vi "configuration UI.vi"() -> ()   [LabVIEW 2013, in "OPC UA Client editor node.lvclass"]
uses:
  OPC UA Client editor node.lvclass
  <vilib>/NI/Configuration Framework/Node/NodeRef.ctl
  <vilib>/NI/Configuration Framework/Node/NISE_CEF_Node.lvclass
  <vilib>/NI/AMC/Message Queue.ctl
  <vilib>/NI/AMC/Message.ctl
  <vilib>/NI/Tools/Keyed Array/KeyedArray.ctl
  <vilib>/NI/Configuration Framework/Node/UserEventRef.ctl
  <vilib>/NI/Configuration Framework/Controls/EventCluster.ctl
  <vilib>/NI/DCAF UI Toolkit/Controls/Configure.ctl
  <vilib>/NI/DCAF UI Toolkit/Controls/Add.ctl
  <vilib>/NI/DCAF UI Toolkit/Controls/Remove.ctl
  <vilib>/NI/Configuration Framework/Node/StopEvent.ctl
  <vilib>/NI/Configuration Framework/Node/RefreshUIEvent.ctl
  <vilib>/NI/Configuration Framework/Node/CacheState.ctl
  <vilib>/NI/Configuration Framework/Node/NodeChangeEvent.ctl
  <vilib>/NI/Tag Bus/tag/Data Type.ctl
  Permissions Enum.ctl
  <vilib>/NI/DCAF/Tag Editor Core/Table API/Available Tag Menu/channel action event.ctl
  <vilib>/NI/DCAF/Tag Editor Core/Table API/Available Tag Menu/dialog output action.ctl
  <vilib>/NI/Tag Bus Module Framework/channel/TBM channel.lvclass
  <vilib>/NI/Tag Bus/tag/tag descriptor.lvclass
  <vilib>/NI/DCAF/Tag Editor Core/Table API/Table Manager/Call Back Ref Type Def.ctl
  <vilib>/NI/DCAF/Tag Editor Core/Configuration Editor/Classes/Engine Parent/Engine Parent Editor Node.lvclass
  OPC UA DataType Enum.ctl
  <vilib>/NI/DCAF/Tag Editor Core/Table API/Table Manager/references.ctl
  module/configuration/OPC UA Client configuration.lvclass
  module/configuration/OPC UA Client configuration.lvclass/OPC UA Client configuration.ctl
  <vilib>/NI/DCAF/Tag Editor Core/Table API/Listbox/Multi Column Listbox.lvclass
  OPC UA Client editor node.lvclass/OPC UA Client editor node.ctl
  module/configuration/Read Connection Configuration.vi
  module/configuration/Write Connection Configuration.vi
  <vilib>/NI/DCAF/Tag Editor Core/Configuration Editor/Classes/Module editor node/module editor node.lvclass
  <vilib>/NI/Configuration Framework/serializable configuration/NISE_CEF_serializable configuration.lvclass
  <vilib>/NI/Configuration Framework/NISE_CEF_TreeControl.lvlib
  <vilib>/NI/Tools/Keyed Array/Tools_KeyedArray.lvlib
  <vilib>/NI/AMC/AMC.lvlib
  <vilib>/NI/DCAF/Tag Editor Core/Table API/Table Manager.lvlib
  <vilib>/NI/DCAF/Tag Editor Core/Table API/Table Manager/Table Manager.lvclass
  <vilib>/NI/DCAF UI Toolkit/Controls/DCAF UI Elements.lvlib
panel:
  in  "OPC Data Type":T1
  in  "user event out":refnum<user-event>
  in  "Permissions":T2
  in  "data type":T3
  in  "node change":T4
  in  "cache state":T5
  in  "refresh UI":T6
  in  "stop event":T7
  in  "Tab Control":enum32{"Nodes", "Client Configuration"}(tab)
  in  "Remove Button":T8
  in  "Add Button":T9
  in  "Table":i32(listbox)
  in  "settings":T10
  in  "Server Certificates":path[](array[path])
  in  "Client Certificate":path
  in  "Server Endpoint URL":string
  in  "Username/Password":cluster{"Username":string, "Password":string}
  in  "Security Policy":T11
  in  "user event":T12
  in  "main queue":T13
  in  "node ref":T14
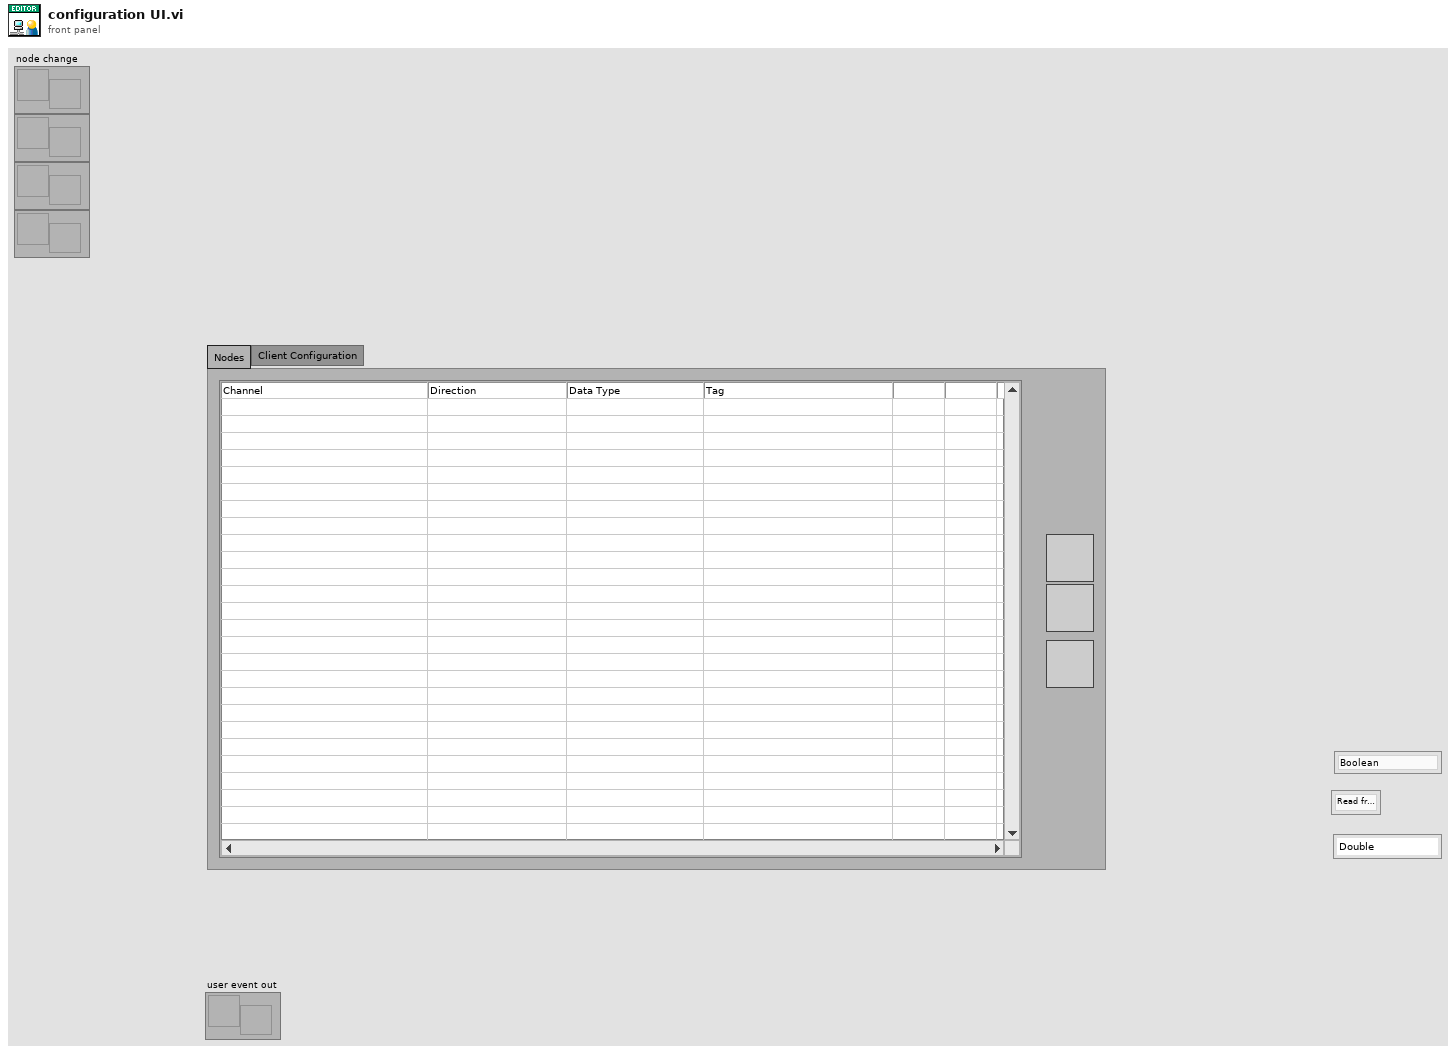
[diagram p1: front panel]
types:
  T1 = typedef "OPC UA Client editor node.lvclass/OPC UA DataType Enum.ctl" = enum16{"Boolean", "SByte", "Byte", "Int16", "UInt16", "Int32", "UInt32", "Int64", "UInt64", "Float", "Double", "String", "DateTime", "ByteString", "Array of Boolean", "Array of SByte", "Array of Byte", "Array of Int16", "Array of UInt16", "Array of Int32", "Array of UInt32", "Array of Int64", "Array of UInt64", "Array of Float", "Array of Double", "Array of String", "Array of DateTime"}
  T2 = typedef "OPC UA Client editor node.lvclass/Permissions Enum.ctl" = enum16{"Read from HW", "Write to HW"}
  T3 = typedef "tag bus.lvlib/tag descriptor.lvclass/Data Type.ctl" = enum16{"Double", "Single", "I64", "I32", "I16", "I8", "U64", "U32", "U16", "U8", "Boolean", "String", "Array of Double", "Array of Single", "Array of I64", "Array of I32", "Array of I16", "Array of I8", "Array of U64", "Array of U32", "Array of U16", "Array of U8", "Array of Boolean", "Array of String"}
  T4 = typedef "NISE_CEF_Node.lvclass/NodeChangeEvent.ctl" = refnum<user-event>
  T5 = typedef "NISE_CEF_Node.lvclass/CacheState.ctl" = refnum<user-event>
  T6 = typedef "NISE_CEF_Node.lvclass/RefreshUIEvent.ctl" = refnum<user-event>
  T7 = typedef "NISE_CEF_Node.lvclass/StopEvent.ctl" = refnum<user-event>
  T8 = typedef "DCAF UI Elements.lvlib/Remove.ctl" = bool
  T9 = typedef "DCAF UI Elements.lvlib/Add.ctl" = bool
  T10 = typedef "DCAF UI Elements.lvlib/Configure.ctl" = bool
  T11 = cluster{"Message Mode":enum16{"None", "Sign", "Sign and Encrypt"}, "Security":enum16{"Basic256", "Basic128Rsa15"}}
  T12 = typedef "NISE_CEF_Node.lvclass/UserEventRef.ctl" = refnum<user-event>
  T13 = typedef "AMC.lvlib/Message Queue.ctl" = refnum<queue>
  T14 = typedef "NISE_CEF_Node.lvclass/NodeRef.ctl" = refnum<data-value>
  T15 = typedef "Table Manager.lvlib/Table Manager.lvclass/references.ctl" = cluster{"stop event":T7, "refresh UI":T6, "cache state":T5, "node change":T4, "user event out":refnum<user-event>, "main queue":T13, "user event":T12}
  T16 = typedef "Table Manager.lvlib/Table Manager.lvclass/object ref.ctl" = cluster{"engine":refnum<data-value>, "Node Ref":refnum<data-value>}
  T17 = cluster{"Server Certificates":cluster{"Relative Path?":bool, "Certificate Paths":path[], "Certificate Names":string[]}, "Client Certificates":cluster{"Relative Path?":bool, "Certificate Paths":path[], "Certificate Names":string[]}, "Client Configuration":cluster{"Server Endpoint URL":string, "Security Policy":cluster{"Message Mode":enum16{"None", "Sign", "Sign and Encrypt"}, "Security":enum16{"Basic256", "Basic128Rsa15"}}, "Username/Password":cluster{"Username":string, "Password":string}}}
  T18 = typedef "Table Manager.lvlib/Column.lvclass/Column Descriptor.ctl" = cluster{"name":string, "caption":string, "Column Type":T19, "Params":string, "AutoSizeMode":i32, "FillWeight":sgl, "MinWidth":u32, "tooltip":string, "Enum Reference":refnum<vi>, "Channel suffix":string, "Read Only":bool, "Call Back VI":T20, "DT Dependency":i32, "name dependency":i32, "data type":T3, "Custom Column":refnum<class "Column.lvclass">}
  T19 = typedef "Table Manager.lvlib/Column.lvclass/Column Type.ctl" = enum16{"String", "Mapping", "Enum", "Custom"}
  T20 = typedef "Table Manager.lvlib/Table Manager.lvclass/Call Back Ref Type Def.ctl" = refnum<vi>
  T21 = typedef "Table Manager.lvlib/Table Manager.lvclass/Table Events.ctl" = cluster{"Menu Selection":refnum<user-event>}
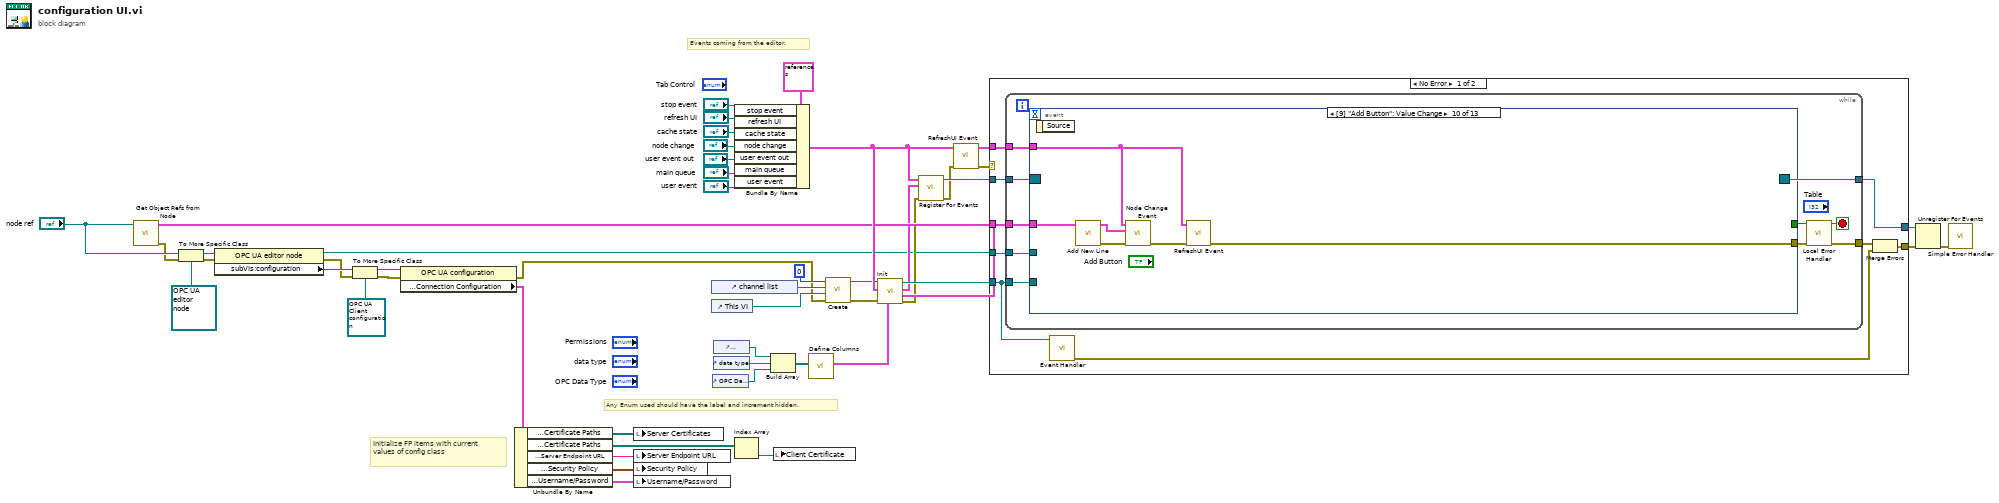
[diagram p0: block diagram]
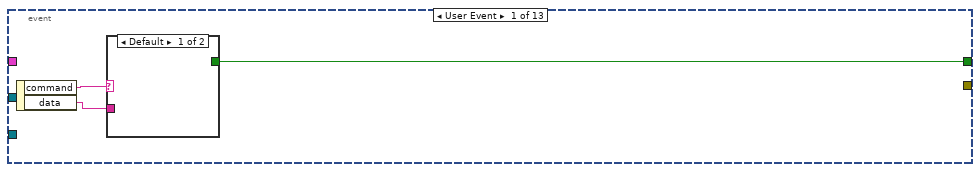
[diagram p2: hidden frame]
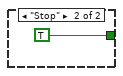
[diagram p3: hidden frame]
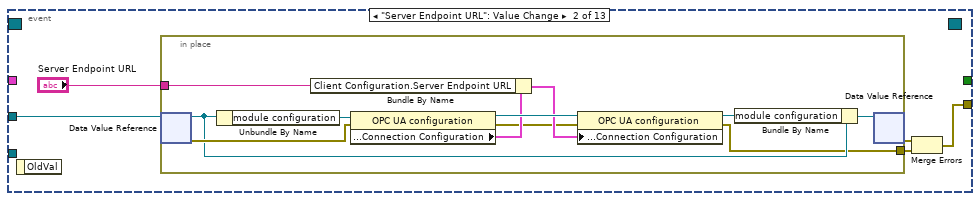
[diagram p4: hidden frame]
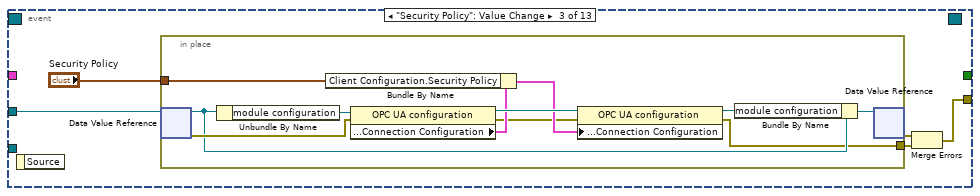
[diagram p5: hidden frame]
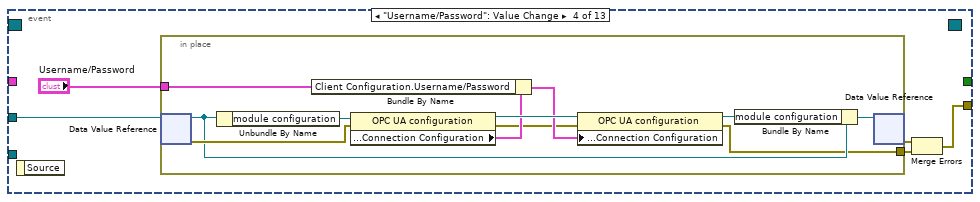
[diagram p6: hidden frame]
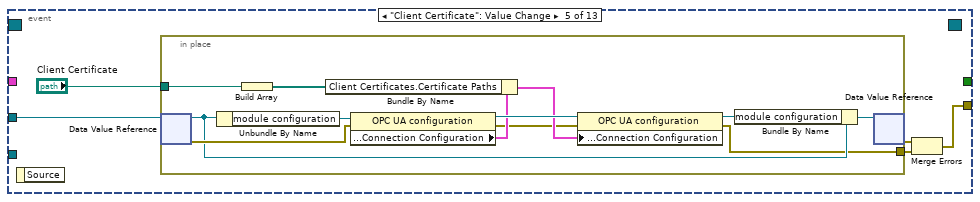
[diagram p7: hidden frame]
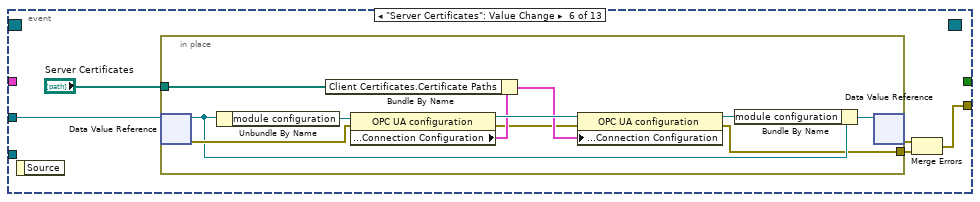
[diagram p8: hidden frame]
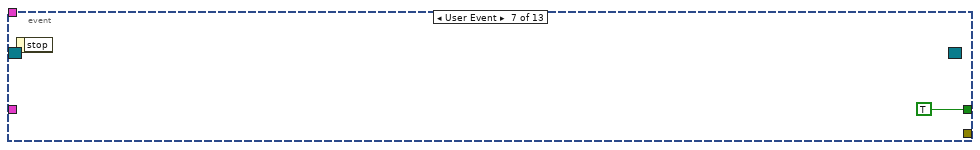
[diagram p9: hidden frame]
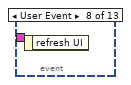
[diagram p10: hidden frame]
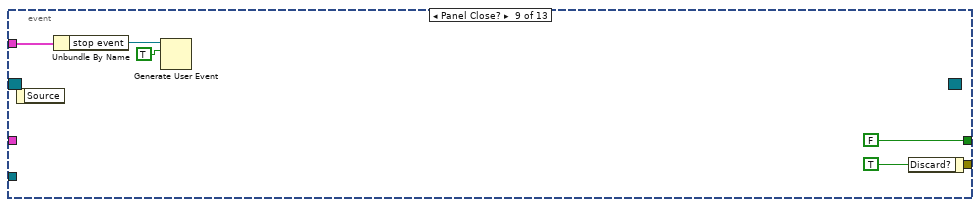
[diagram p11: hidden frame]
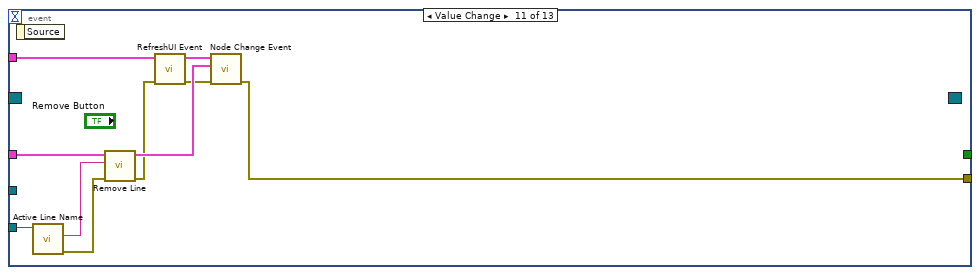
[diagram p12: hidden frame]
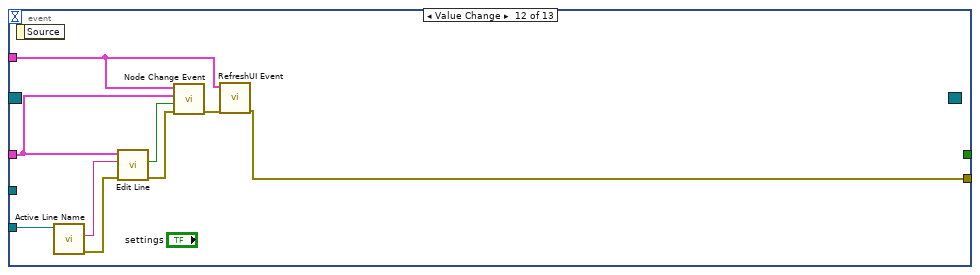
[diagram p13: hidden frame]
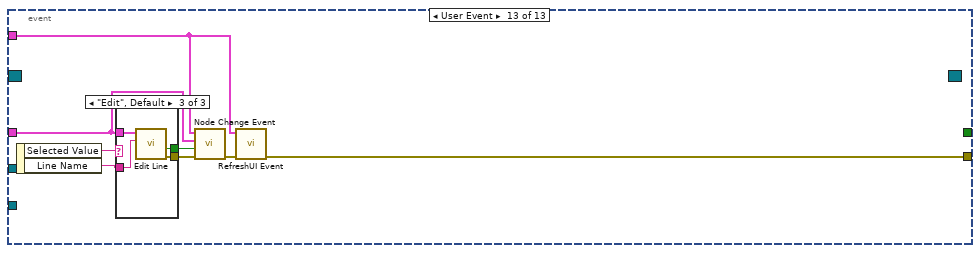
[diagram p14: hidden frame]
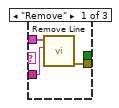
[diagram p15: hidden frame]
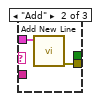
[diagram p16: hidden frame]
diagram:
  # "Initialize FP items with current values of config class"
  # "Any Enum used should have the label and increment hidden."
  # "Events coming from the editor."
  n1 = call "Get Object Refs from Node.vi"("Data Value Reference in"="node ref") -> ("error out"=w18:errorcluster, "references"=w32:T16)  [unwired: 9 in]
  n2 = To More Specific Class(target class=refnum<data-value> refnum ("data value reference"), reference="node ref", error in=w18) -> (specific class reference=w16:refnum<data-value>, error out=w17:errorcluster)
  n3 = property class="OPC UA editor node"(reference=w16, error in=w17) -> (reference out=w15:refnum<data-value>, error out=w9:errorcluster, "subVIs:configuration"=w14:refnum<class "NISE_CEF_serializable configuration.lvclass">)
  n4 = To More Specific Class(target class=refnum<class "OPC UA Client configuration.lvclass"> refnum ("OPC UA configuration"), reference=w14, error in=w9) -> (specific class reference=w13:refnum<class "OPC UA Client configuration.lvclass">, error out=w12:errorcluster)
  n5 = property class="OPC UA configuration"(reference=w13, error in=w12) -> (error out=w8:errorcluster, "Customize:Properties:Connection Configuration"=w10:T17)  [unwired: 1 out]
  n6 = Unbundle By Name(w10) -> ("Server Certificates.Certificate Paths"=w6:path[], "Client Certificates.Certificate Paths"=w5:path[], "Client Configuration.Server Endpoint URL"=w1:string, "Client Configuration.Security Policy"=w2:T11, "Client Configuration.Username/Password"=w3:cluster{"Username":string, "Password":string})
  n7 = local write "Server Certificates"(w6) -> ()
  n8 = local write "Server Endpoint URL"(w1) -> ()
  n9 = local write "Security Policy"(w2) -> ()
  n10 = local write "Username/Password"(w3) -> ()
  n11 = control-ref of="channel list"() -> (w25:refnum<vi>)
  n12 = control-ref of="This VI"() -> (w23:refnum<vi>)
  n13 = control-ref of="OPC Data Type"() -> (w21:refnum<vi>)
  n14 = control-ref of="Permissions"() -> (w35:refnum<vi>)
  n15 = control-ref of="data type"() -> (w34:refnum<vi>)
  n16 = Bundle By Name(cluster=T15 {"stop event"=refnum, "refresh UI"=refnum, "cache state"=refnum, "node change"=refnum, "user event out"=refnum, "main queue"=refnum, "user event"=refnum} ("References"), "stop event"="stop event", "refresh UI"="refresh UI", "cache state"="cache state", "node change"="node change", "user event out"="user event out", "main queue"="main queue", "user event"="user event") -> (w36:T15)
  n17 = Index Array(array=w5) -> (element=w4:path)  [unwired: 1 in]
  n18 = Build Array(w35, w34, w21) -> (w33:refnum<vi>[])
  n19 = local write "Client Certificate"(w4) -> ()
  n20 = call "Define Columns.vi"("Enum Array"=w33) -> ("Column Definition"=w38:T18[])  [unwired: 10 in]
  n21 = call <vilib>:"Create.vi"("error in (no error)"=w8, "Top VI"=w23, "Listbox"=w25, "Index"=0) -> ("error out"=w7:errorcluster, "reference out"=w22:refnum<class "Multi Column Listbox.lvclass">)  [unwired: 6 in]
  n22 = call-dynamic "Init.vi"("Column Descriptors"=w38, "error in (no error)"=w7, "Node object refs"=w32, "Event References"=w36, "Multi Column Listbox in"=w22) -> ("error out"=w27:errorcluster, "Table Events"=w26:T21, "Multi Column Listbox out"=w31:refnum<class "Multi Column Listbox.lvclass">)  [unwired: 4 in]
  n23 = call "Register For Events.vi"("error in"=w27, "Table Events"=w26, "References"=w36) -> ("error out"=w29:errorcluster, "Event Registration Refnum"=w39:refnum<event-registration>)  [unwired: 7 in]
  n24 = call "RefreshUI Event.vi"("error in (no error)"=w29, "References in"=w36) -> ("error out"=w28:errorcluster, "References out"=w37:T15)  [unwired: 8 in]
  n25 = case shown="No Error" w28 {
    selector: w28 -> [_ w201]
    tunnel: w39 -> [w58 w200]
    tunnel: [w57 w200] -> w49
    tunnel: [w51 w201] -> w48
    tunnel: w37 -> [w56 _]
    tunnel: w32 -> [w55 _]
    tunnel: w31 -> [w54 _]
    tunnel: w15 -> [w50 _]
    frame No Error {
      n26 = while {
        tunnel: w58 -> [w68]
        tunnel: [w67] -> w57
        tunnel: [w64] -> w52
        tunnel: w56 -> [w62]
        tunnel: w55 -> [w61]
        tunnel: w54 -> [w60]
        tunnel: w50 -> [w59]
        stop <- w66 stop-if-true
        n27 = event shown="[9] \"Add Button\": Value Change" {
          selector: w68 -> [_ _ _ _ _ _ _ _ _ _ _ _ _]
          dyn-events: [_ _ _ _ _ _ _ _ _ _ _ _ _] -> w67
          timeout: _ -> [_ _ _ _ _ _ _ _ _ _ _ _ _]
          tunnel: [w71 _ _ _ _ _ TRUE _ FALSE _ _ _ _] -> w65
          tunnel: [_ w73 w90 w106 w122 w139 _ _ _ w160 w168 w175 w188] -> w63
          tunnel: w62 -> [_ _ _ _ _ _ _ _ w156 w163 w173 w174 w184]
          tunnel: w61 -> [_ _ _ _ _ _ _ _ _ w164 w172 w180 w185]
          tunnel: w60 -> [_ _ _ _ _ _ _ _ _ _ w167 w181 _]
          tunnel: w59 -> [_ w77 w93 w109 w125 w142 _ _ _ _ _ _ _]
          event User Event {
            n28 = event-data() -> ("command"=w70:string, "data"=w69:string)  [unwired: 1 in]
            n29 = case shown="Default" w70 {
              tunnel: [_ TRUE] -> w71
              tunnel: w69 -> [_ _]
              frame Default {
              }
              frame "Stop" {
              }
            }
          }
          event "Server Endpoint URL": Value Change {
            n30 = event-data() -> ()  [unwired: 1 in, 1 out]
            n31 = in-place {
              in-place-border: "Server Endpoint URL" -> [w84]
              in-place-border: [w78] -> w74
              n32 = in-place-dvr #1(w77) -> (w80:refnum<class "OPC UA Client editor node.lvclass">, w83:errorcluster)
              n33 = Unbundle By Name(w80) -> ("module configuration"=w88:refnum<class "OPC UA Client configuration.lvclass">)
              n34 = property class="OPC UA configuration"(reference=w88, error in=w83) -> (reference out=w87:refnum<class "OPC UA Client configuration.lvclass">, error out=w82:errorcluster, "Customize:Properties:Connection Configuration"=w86:T17)
              n35 = Bundle By Name(cluster=w86, "Client Configuration.Server Endpoint URL"=w84) -> (w85:T17)
              n36 = property class="OPC UA configuration"(reference=w87, error in=w82, "Customize:Properties:Connection Configuration"=w85) -> (reference out=w81:refnum<class "OPC UA Client configuration.lvclass">, error out=w78:errorcluster)
              n37 = Bundle By Name(cluster=w80, "module configuration"=w81) -> (w79:refnum<class "OPC UA Client editor node.lvclass">)
              n38 = in-place-dvr #1(w79) -> (w75:errorcluster)  [unwired: 1 out]
            }
            n39 = Merge Errors(w75, w74) -> (w73:errorcluster)
          }
          event "Security Policy": Value Change {
            n40 = event-data() -> ()  [unwired: 1 in, 1 out]
            n41 = in-place {
              in-place-border: "Security Policy" -> [w100]
              in-place-border: [w94] -> w91
              n42 = in-place-dvr #2(w93) -> (w96:refnum<class "OPC UA Client editor node.lvclass">, w99:errorcluster)
              n43 = Unbundle By Name(w96) -> ("module configuration"=w104:refnum<class "OPC UA Client configuration.lvclass">)
              n44 = property class="OPC UA configuration"(reference=w104, error in=w99) -> (reference out=w103:refnum<class "OPC UA Client configuration.lvclass">, error out=w98:errorcluster, "Customize:Properties:Connection Configuration"=w102:T17)
              n45 = Bundle By Name(cluster=w102, "Client Configuration.Security Policy"=w100) -> (w101:T17)
              n46 = property class="OPC UA configuration"(reference=w103, error in=w98, "Customize:Properties:Connection Configuration"=w101) -> (reference out=w97:refnum<class "OPC UA Client configuration.lvclass">, error out=w94:errorcluster)
              n47 = Bundle By Name(cluster=w96, "module configuration"=w97) -> (w95:refnum<class "OPC UA Client editor node.lvclass">)
              n48 = in-place-dvr #2(w95) -> (w92:errorcluster)  [unwired: 1 out]
            }
            n49 = Merge Errors(w92, w91) -> (w90:errorcluster)
          }
          event "Username/Password": Value Change {
            n50 = event-data() -> ()  [unwired: 1 in, 1 out]
            n51 = in-place {
              in-place-border: "Username/Password" -> [w116]
              in-place-border: [w110] -> w107
              n52 = in-place-dvr #3(w109) -> (w112:refnum<class "OPC UA Client editor node.lvclass">, w115:errorcluster)
              n53 = Unbundle By Name(w112) -> ("module configuration"=w120:refnum<class "OPC UA Client configuration.lvclass">)
              n54 = property class="OPC UA configuration"(reference=w120, error in=w115) -> (reference out=w119:refnum<class "OPC UA Client configuration.lvclass">, error out=w114:errorcluster, "Customize:Properties:Connection Configuration"=w118:T17)
              n55 = Bundle By Name(cluster=w118, "Client Configuration.Username/Password"=w116) -> (w117:T17)
              n56 = property class="OPC UA configuration"(reference=w119, error in=w114, "Customize:Properties:Connection Configuration"=w117) -> (reference out=w113:refnum<class "OPC UA Client configuration.lvclass">, error out=w110:errorcluster)
              n57 = Bundle By Name(cluster=w112, "module configuration"=w113) -> (w111:refnum<class "OPC UA Client editor node.lvclass">)
              n58 = in-place-dvr #3(w111) -> (w108:errorcluster)  [unwired: 1 out]
            }
            n59 = Merge Errors(w108, w107) -> (w106:errorcluster)
          }
          event "Client Certificate": Value Change {
            n60 = event-data() -> ()  [unwired: 1 in, 1 out]
            n61 = in-place {
              in-place-border: "Client Certificate" -> [w133]
              in-place-border: [w127] -> w123
              n62 = in-place-dvr #4(w125) -> (w129:refnum<class "OPC UA Client editor node.lvclass">, w132:errorcluster)
              n63 = Unbundle By Name(w129) -> ("module configuration"=w137:refnum<class "OPC UA Client configuration.lvclass">)
              n64 = Build Array(w133) -> (w126:path[])
              n65 = property class="OPC UA configuration"(reference=w137, error in=w132) -> (reference out=w136:refnum<class "OPC UA Client configuration.lvclass">, error out=w131:errorcluster, "Customize:Properties:Connection Configuration"=w135:T17)
              n66 = Bundle By Name(cluster=w135, "Client Certificates.Certificate Paths"=w126) -> (w134:T17)
              n67 = property class="OPC UA configuration"(reference=w136, error in=w131, "Customize:Properties:Connection Configuration"=w134) -> (reference out=w130:refnum<class "OPC UA Client configuration.lvclass">, error out=w127:errorcluster)
              n68 = Bundle By Name(cluster=w129, "module configuration"=w130) -> (w128:refnum<class "OPC UA Client editor node.lvclass">)
              n69 = in-place-dvr #4(w128) -> (w124:errorcluster)  [unwired: 1 out]
            }
            n70 = Merge Errors(w124, w123) -> (w122:errorcluster)
          }
          event "Server Certificates": Value Change {
            n71 = event-data() -> ()  [unwired: 1 in, 1 out]
            n72 = in-place {
              in-place-border: "Server Certificates" -> [w149]
              in-place-border: [w143] -> w140
              n73 = in-place-dvr #5(w142) -> (w145:refnum<class "OPC UA Client editor node.lvclass">, w148:errorcluster)
              n74 = Unbundle By Name(w145) -> ("module configuration"=w153:refnum<class "OPC UA Client configuration.lvclass">)
              n75 = property class="OPC UA configuration"(reference=w153, error in=w148) -> (reference out=w152:refnum<class "OPC UA Client configuration.lvclass">, error out=w147:errorcluster, "Customize:Properties:Connection Configuration"=w151:T17)
              n76 = Bundle By Name(cluster=w151, "Client Certificates.Certificate Paths"=w149) -> (w150:T17)
              n77 = property class="OPC UA configuration"(reference=w152, error in=w147, "Customize:Properties:Connection Configuration"=w150) -> (reference out=w146:refnum<class "OPC UA Client configuration.lvclass">, error out=w143:errorcluster)
              n78 = Bundle By Name(cluster=w145, "module configuration"=w146) -> (w144:refnum<class "OPC UA Client editor node.lvclass">)
              n79 = in-place-dvr #5(w144) -> (w141:errorcluster)  [unwired: 1 out]
            }
            n80 = Merge Errors(w141, w140) -> (w139:errorcluster)
          }
          event User Event {
            n81 = event-data() -> ()  [unwired: 1 in, 1 out]
          }
          event User Event {
            n82 = event-data() -> ()  [unwired: 1 in, 1 out]
          }
          event Panel Close? {
            n83 = event-data() -> ()  [unwired: 1 in, 1 out]
            n84 = Unbundle By Name(w156) -> ("stop event"=w155:T7)
            n85 = Generate User Event(user event=w155, event data cluster=TRUE ("event data")) -> ()  [unwired: 2 in, 2 out]
            n86 = event-data("Discard?"=TRUE) -> ()  [unwired: 1 in, 1 out]
          }
          event Value Change {
            n87 = event-data() -> ()  [unwired: 1 in, 1 out]
            n88 = call "Add New Line.vi"("objects"=w164) -> ("error out"=w162:errorcluster)  [unwired: 9 in, 1 out]
            n89 = call "Node Change Event.vi"("error in (no error)"=w162, "objects"=w164, "References in"=w163) -> ("error out"=w161:errorcluster)  [unwired: 8 in]
            n90 = call "RefreshUI Event.vi"("error in (no error)"=w161, "References in"=w163) -> ("error out"=w160:errorcluster)  [unwired: 8 in, 1 out]
          }
          event Value Change {
            n91 = event-data() -> ()  [unwired: 1 in, 1 out]
            n92 = call-dynamic "Active Line Name.vi"("Multi Column Listbox in"=w167) -> ("error out"=w165:errorcluster, "Active Line Name"=w166:string)  [unwired: 8 in, 1 out]
            n93 = call "Remove Line.vi"("error in"=w165, "Active Line Name"=w166, "Objects"=w172) -> ("error out"=w169:errorcluster)  [unwired: 8 in]
            n94 = call "RefreshUI Event.vi"("error in (no error)"=w169, "References in"=w173) -> ("error out"=w171:errorcluster, "References out"=w170:T15)  [unwired: 8 in]
            n95 = call "Node Change Event.vi"("error in (no error)"=w171, "objects"=w172, "References in"=w170) -> ("error out"=w168:errorcluster)  [unwired: 8 in]
          }
          event Value Change {
            n96 = event-data() -> ()  [unwired: 1 in, 1 out]
            n97 = call-dynamic "Active Line Name.vi"("Multi Column Listbox in"=w181) -> ("error out"=w178:errorcluster, "Active Line Name"=w179:string)  [unwired: 8 in, 1 out]
            n98 = call "Edit Line.vi"("error in"=w178, "Line Name"=w179, "References"=w180) -> ("error out"=w182:errorcluster, "change?"=w177:bool)  [unwired: 7 in]
            n99 = call "Node Change Event.vi"("error in (no error)"=w182, "Send"=w177, "objects"=w180, "References in"=w174) -> ("error out"=w176:errorcluster)  [unwired: 7 in]
            n100 = call "RefreshUI Event.vi"("error in (no error)"=w176, "References in"=w174) -> ("error out"=w175:errorcluster)  [unwired: 8 in, 1 out]
          }
          event User Event {
            n101 = event-data() -> ("Selected Value"=w190:string, "Line Name"=w187:string)  [unwired: 1 in]
            n102 = case shown="\"Edit\", Default" w190 {
              tunnel: w187 -> [w193 _ w199]
              tunnel: w185 -> [w192 w195 w198]
              tunnel: [w191 w194 w197] -> w186
              tunnel: [_ _ w196] -> w183
              frame "Remove" {
                n103 = call "Remove Line.vi"("Active Line Name"=w193, "Objects"=w192) -> ("error out"=w191:errorcluster)  [unwired: 9 in]
              }
              frame "Add" {
                n104 = call "Add New Line.vi"("objects"=w195) -> ("error out"=w194:errorcluster)  [unwired: 9 in, 1 out]
              }
              frame "Edit", Default {
                n105 = call "Edit Line.vi"("Line Name"=w199, "References"=w198) -> ("error out"=w197:errorcluster, "change?"=w196:bool)  [unwired: 8 in]
              }
            }
            n106 = call "Node Change Event.vi"("error in (no error)"=w186, "Send"=w183, "objects"=w185, "References in"=w184) -> ("error out"=w189:errorcluster)  [unwired: 7 in]
            n107 = call "RefreshUI Event.vi"("error in (no error)"=w189, "References in"=w184) -> ("error out"=w188:errorcluster)  [unwired: 8 in, 1 out]
          }
        }
        n108 = call "Local Error Handler.vi"("error in"=w63, "Stop in"=w65) -> ("error out"=w64:errorcluster, "Stop out"=w66:bool)  [unwired: 8 in]
      }
      n109 = call-dynamic "Event Handler.vi"("Listbox in"=w54) -> ("error out"=w53:errorcluster)  [unwired: 9 in, 1 out]
      n110 = Merge Errors(w52, w53) -> (w51:errorcluster)
    }
    frame Error {
    }
  }
  n111 = Unregister For Events(event registration refnum=w49, error in=w48) -> (error out=w47:errorcluster)
  n112 = call <vilib>:"Simple Error Handler.vi"("error in (no error)"=w47) -> ()  [unwired: 4 in, 5 out]
